vi "Capture@Snap__Parameter.vi"(1 "ParamterIn":string) -> (0 "ParamterOut":string)   [LabVIEW 2020]
panel:
  in  "Message":string(combo)
  in  "IMAQName":string(combo)
  in  "CamName":string(combo)
  in  "Confirm":bool
  # "Capture@Snap $Capture(,$ImaqName,[[$label]]$Message)"
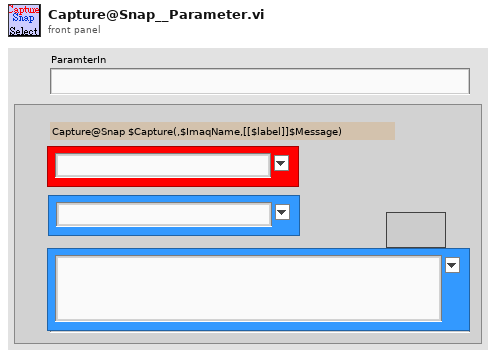
[diagram p1: front panel]
types:
  T1 = enum16{"Get", "Get&Index+1", "Insert", "Init", "Clear", "SetIndex"}
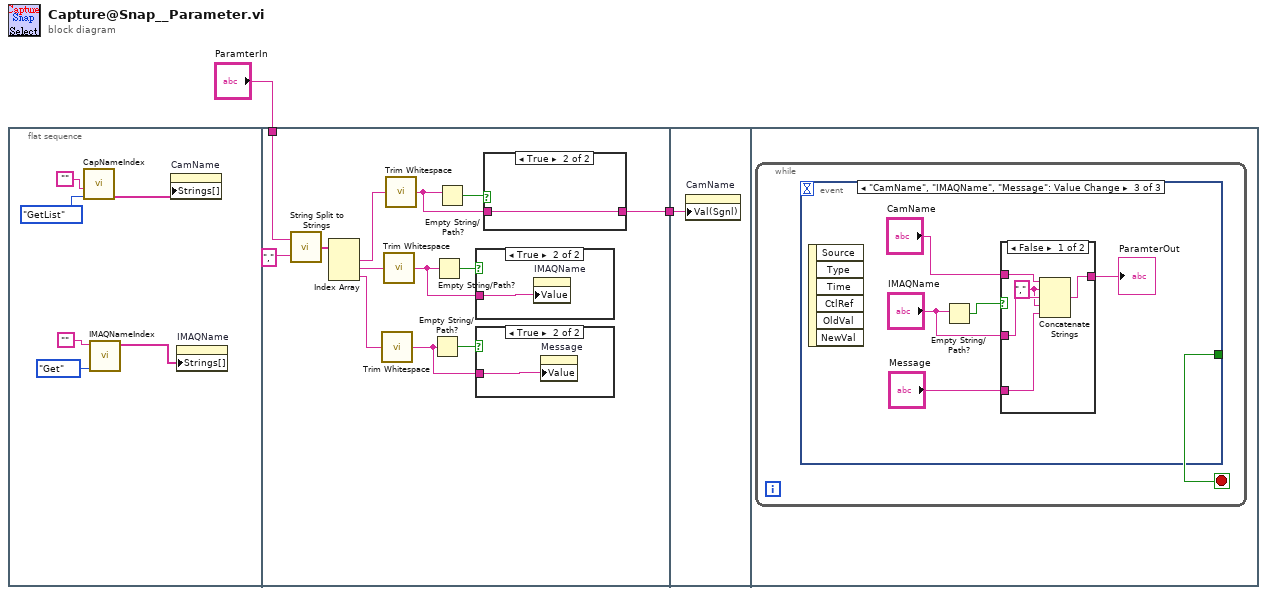
[diagram p0: block diagram]
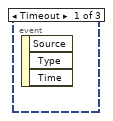
[diagram p5: hidden frame]
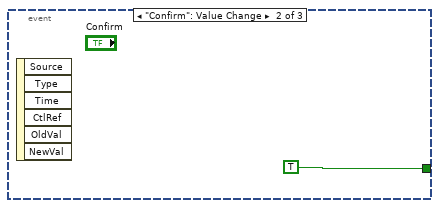
[diagram p6: hidden frame]
diagram:
  n1 = flat-sequence {
    tunnel: "ParamterIn" -> [w14]
    tunnel: [w17] -> w1
    tunnel: w1 -> [w26]
    frame #0 {
      n2 = call "CapNameIndex.vi"("OP"=enum16{"AddCam", "GetIndex", "Init", "GetList"}."GetList", "CamName"="") -> ("DeviceList"=w7:string[])  [unwired: 2 in, 3 out]
      n3 = call "IMAQNameIndex.vi"("OP"=T1."Get", "IMAQName"="") -> ("IMAQNameList"=w3:string[])  [unwired: 2 in, 7 out]
      n4 = property on="CamName" class="CmbBox"("Strings[]"=w7) -> ()  [unwired: 2 in, 2 out]
      n5 = property on="IMAQName" class="CmbBox"("Strings[]"=w3) -> ()  [unwired: 2 in, 2 out]
    }
    frame #1 {
      n6 = call "String Split to Strings.vi"("search string/char (-)"=",", "String"=w14) -> ("Array"=w16:string[])
      n7 = Index Array(array=w16) -> (element #1=w13:string, element #2=w12:string, element #3=w11:string)  [unwired: 3 in]
      n8 = call <vilib>:"Trim Whitespace.vi"("string"=w11) -> ("trimmed string"=w9:string)  [unwired: 1 in]
      n9 = call <vilib>:"Trim Whitespace.vi"("string"=w12) -> ("trimmed string"=w18:string)  [unwired: 1 in]
      n10 = call <vilib>:"Trim Whitespace.vi"("string"=w13) -> ("trimmed string"=w20:string)  [unwired: 1 in]
      n11 = Empty String/Path?(string/path=w9) -> (empty?=w10:bool)
      n12 = Empty String/Path?(string/path=w18) -> (empty?=w19:bool)
      n13 = Empty String/Path?(string/path=w20) -> (empty?=w21:bool)
      n14 = case shown="True" w19 {
        tunnel: w18 -> [_ w23]
        frame False {
        }
        frame True {
          n15 = property on="IMAQName" class="CmbBox"("Value"=w23) -> ()  [unwired: 2 in, 2 out]
        }
      }
      n16 = case shown="True" w10 {
        tunnel: w9 -> [_ w22]
        frame False {
        }
        frame True {
          n17 = property on="Message" class="CmbBox"("Value"=w22) -> ()  [unwired: 2 in, 2 out]
        }
      }
      n18 = case shown="True" w21 {
        tunnel: w20 -> [w24 w25]
        tunnel: [w24 w25] -> w17
        frame False {
        }
        frame True {
        }
      }
    }
    frame #2 {
      n19 = property on="CamName" class="CmbBox"("Val(Sgnl)"=w26) -> ()  [unwired: 2 in, 2 out]
    }
    frame #3 {
      n20 = while {
        stop <- w27 stop-if-true
        n21 = event shown="[2] \"CamName\", \"IMAQName\", \"Message\": Value Change" {
          selector: _ -> [_ _ _]
          dyn-events: _ -> [_ _ _]
          timeout: _ -> [_ _ _]
          tunnel: [_ TRUE _] -> w27
          event Timeout {
            n22 = event-data() -> ()  [unwired: 1 in, 3 out]
          }
          event "Confirm": Value Change {
            n23 = event-data() -> ()  [unwired: 1 in, 6 out]
          }
          event "CamName", "IMAQName", "Message": Value Change {
            n24 = event-data() -> ()  [unwired: 1 in, 6 out]
            n25 = Empty String/Path?(string/path="IMAQName") -> (empty?=w33:bool)
            n26 = case shown="False" w33 {
              tunnel: [w36 w39] -> w31
              tunnel: "CamName" -> [w38 w39]
              tunnel: "IMAQName" -> [w37 _]
              tunnel: "Message" -> [w34 _]
              frame False {
                w35 = "," ("string")
                n27 = Concatenate Strings(w38, w35, w37, w35, w34) -> (w36:string)
              }
              frame True {
              }
            }
            "ParamterOut" <- w31
          }
        }
      }
    }
  }
